vi "Init.vi"(8 "error in (no error)":errorcluster) -> (0 "error out":errorcluster, 3 "InfoService out":refnum<class "InfoService.lvclass">)   [LabVIEW 2020, in "Vecto.lvlib" / "InfoService.lvclass"]
uses:
  InfoService.lvclass
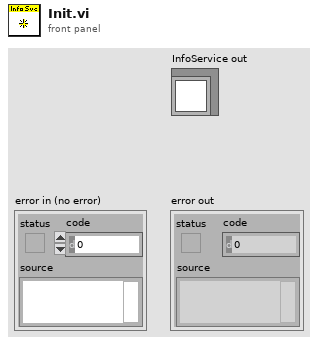
[diagram p1: front panel]
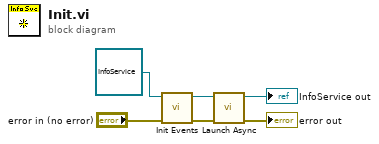
[diagram p0: block diagram]
diagram:
  n1 = call "Init Events.vi"("error in (no error)"="error in (no error)", "InfoService in"=refnum<class "InfoService.lvclass"> refnum) -> ("error out"=w5:errorcluster, "InfoService out"=w2:refnum<class "InfoService.lvclass">)  [unwired: 8 in]
  n2 = call "Launch Async.vi"("error in (no error)"=w5, "InfoService in"=w2) -> ("error out"=→"error out":errorcluster, "InfoService out"=→"InfoService out":refnum<class "InfoService.lvclass">)  [unwired: 8 in]
